vi "JSON Type.vi"(0 "JSON Value":string) -> (1 "JSON Value Type":T1, 2 "JSON Value Out (dup)":string)   [LabVIEW 2011, in "LV JSON.lvlib"]
doc: "Determine the type of JSON object by the first non-whitespace character of the JSON Value.\n\n{\"key\":value}"
uses:
  LV JSON.lvlib
  controls/JSON type.ctl
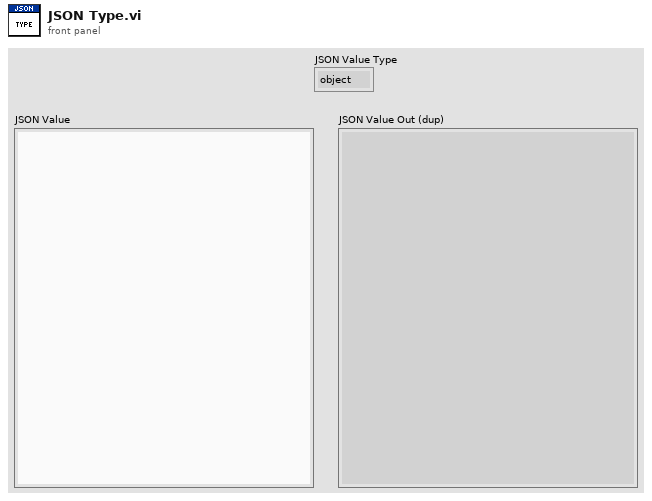
[diagram p1: front panel]
types:
  T1 = typedef "LV JSON.lvlib/JSON type.ctl" = enum16{"object", "array", "number", "string", "boolean", "null"}
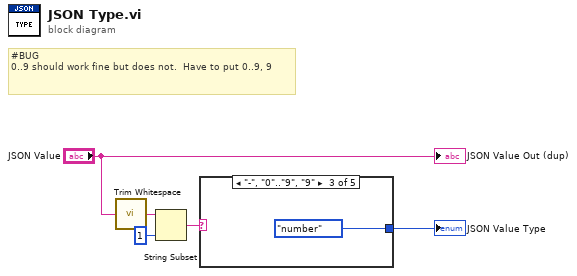
[diagram p0: block diagram]
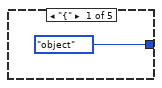
[diagram p2: hidden frame]
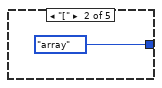
[diagram p3: hidden frame]
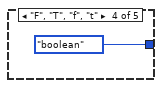
[diagram p4: hidden frame]
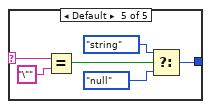
[diagram p5: hidden frame]
diagram:
  # "#BUG\n0..9 should work fine but does not.  Have to put 0..9, 9"
  n1 = call <vilib>:"Trim Whitespace.vi"("string"="JSON Value") -> ("trimmed string"=w1:string)  [unwired: 1 in]
  n2 = String Subset(string=w1, length (rest)=1 ("length (rest)")) -> (substring=w5:string)  [unwired: 1 in]
  n3 = case shown="\"-\", \"0\"..\"9\", \"9\"" w5 {
    selector: w5 -> [_ _ _ _ w14]
    tunnel: [JSON_type."object" ("JSON type") JSON_type."array" ("JSON type") JSON_type."number" ("JSON type") JSON_type."boolean" ("JSON type") w10] -> w3
    frame "{" {
    }
    frame "[" {
    }
    frame "-", "0".."9", "9" {
    }
    frame "F", "T", "f", "t" {
    }
    frame Default {
      n4 = Equal?(x=w14, y="\"") -> (x = y?=w12:bool)
      n5 = Select(t=JSON_type."string" ("JSON type"), s=w12, f=JSON_type."null" ("JSON type")) -> (s? t:f=w10:T1)
    }
  }
  "JSON Value Type" <- w3
  "JSON Value Out (dup)" <- "JSON Value"
